vi "Read Byte.vi"(8 "error in":errorcluster, 11 "File Ref In":refnum<file>) -> (0 "error out":errorcluster, 2 "Word":u8, 3 "File Ref Out":refnum<file>)   [LabVIEW 2020]
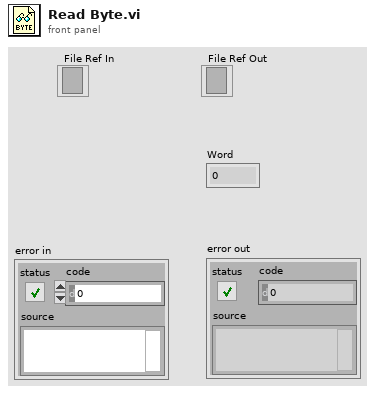
[diagram p1: front panel]
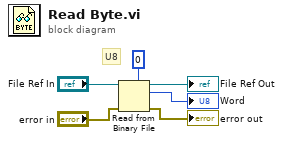
[diagram p0: block diagram]
diagram:
  # "U8"
  n1 = Read from Binary File(5:u8 0, 8:"error in", 11:"File Ref In") -> (0:→"error out":errorcluster, 2:→"Word":u8, 3:→"File Ref Out":refnum<file>)  [unwired: 3 in, 1 out]
